vi "LB_GetHSI.vi"(8 "error in (no error)":errorcluster caption="错误输入（无错误）", 10 "CH":u8=1 min=1, 11 "LB_COM_IN":refnum<visa-resource-name>="COM4") -> (0 "error out":errorcluster caption="错误输出", 1 "Sat":i32, 2 "Hue":dbl, 3 "LB_COM_OUT":refnum<visa-resource-name>, 4 "Lightness":i32, 5 "OK":bool)   [LabVIEW 2015, in "LBAnalyser.lvlib"]
uses:
  LBAnalyser.lvlib
  UartCOM/UARTCOM.lvlib
panel:
  out "读取字符串":string
  # ">=1"
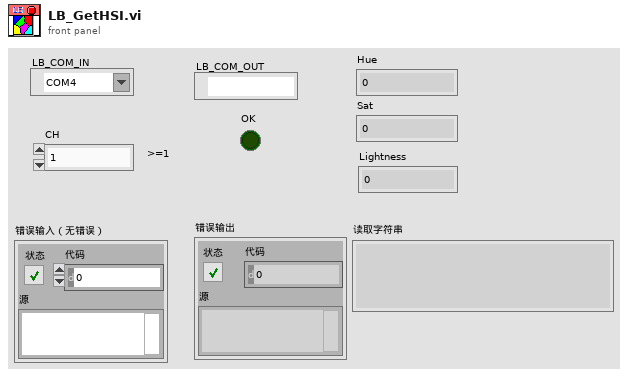
[diagram p1: front panel]
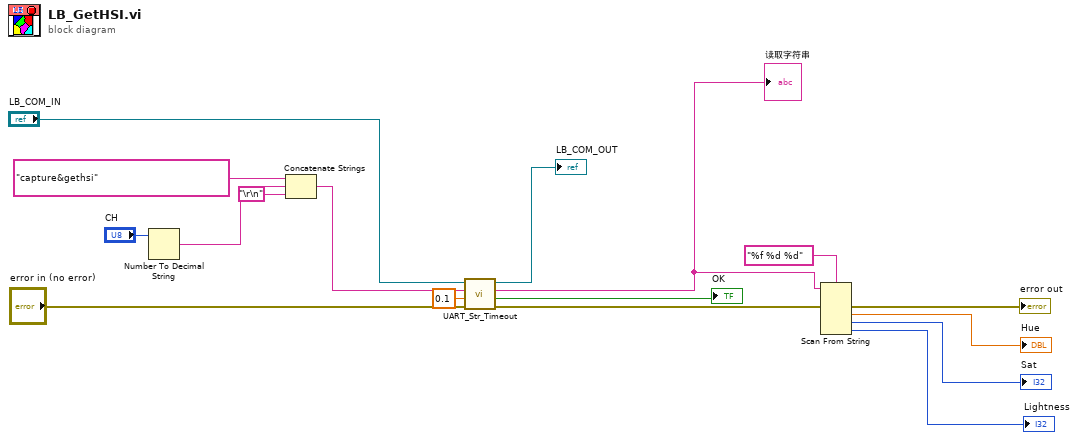
[diagram p0: block diagram]
diagram:
  n1 = Number To Decimal String(number="CH") -> (decimal integer string=w13:string)  [unwired: 1 in]
  n2 = Concatenate Strings("capture&gethsi" ("写入字符串"), w13, "\r\n") -> (w11:string)
  n3 = call "UART_Str_Timeout.vi"("error in (no error)"="error in (no error)", "超时s"=0.1, "写入字符串"=w11, "BASE_COM"="LB_COM_IN") -> ("error out"=w7:errorcluster, "OK"=→"OK":bool, "读取字符串"=w6:string, "BASE_COM_OUT"=→"LB_COM_OUT":refnum<visa-resource-name>)  [unwired: 3 in, 1 out]
  "读取字符串" <- w6
  n4 = Scan From String(format string="%f %d %d" ("格式字符串"), input string=w6, error in=w7) -> (error out=→"error out":errorcluster, output 1=→"Hue":dbl, output 2=→"Sat":i32, output 3=→"Lightness":i32)  [unwired: 4 in, 2 out]
